vi "Color Threshold Handler.vi"(8 "error in (no error)":errorcluster, 11 "Range Updater Cntrl in":T1) -> (0 "error out":errorcluster, 3 "Range Updater Cntrl out":T1)   [LabVIEW 2018]
uses:
  Shared Controls/Range Updater.ctl
  Shared Controls/Threshold Updater.ctl
  Val Change Checker.vi
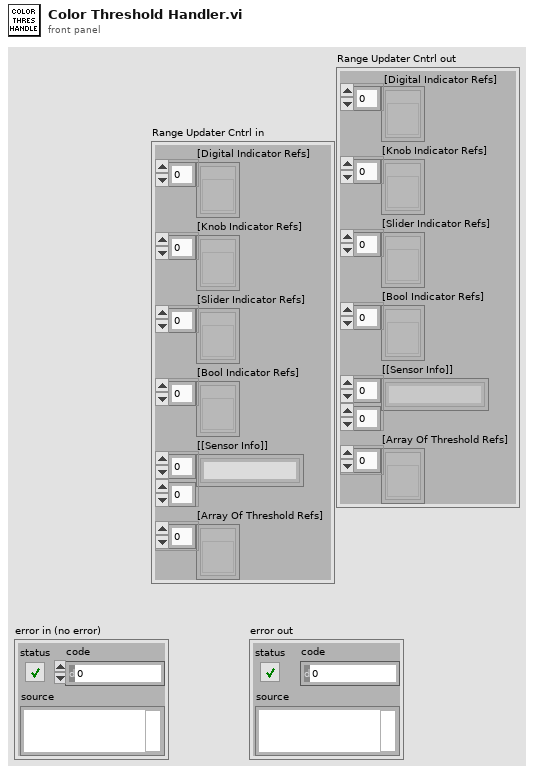
[diagram p1: front panel]
types:
  T1 = typedef "Range Updater.ctl" = cluster{"[Digital Indicator Refs]":refnum<vi>[], "[Knob Indicator Refs]":refnum<vi>[], "[Slider Indicator Refs]":refnum<vi>[], "[Bool Indicator Refs]":refnum<vi>[], "[[Sensor Info]]":string[][], "[Array Of Threshold Refs]":refnum<vi>[]}
  T2 = typedef "Threshold Updater.ctl" = cluster{"Red Min":dbl, "Yellow Min":dbl, "Yellow Max":dbl, "Red Max":dbl}
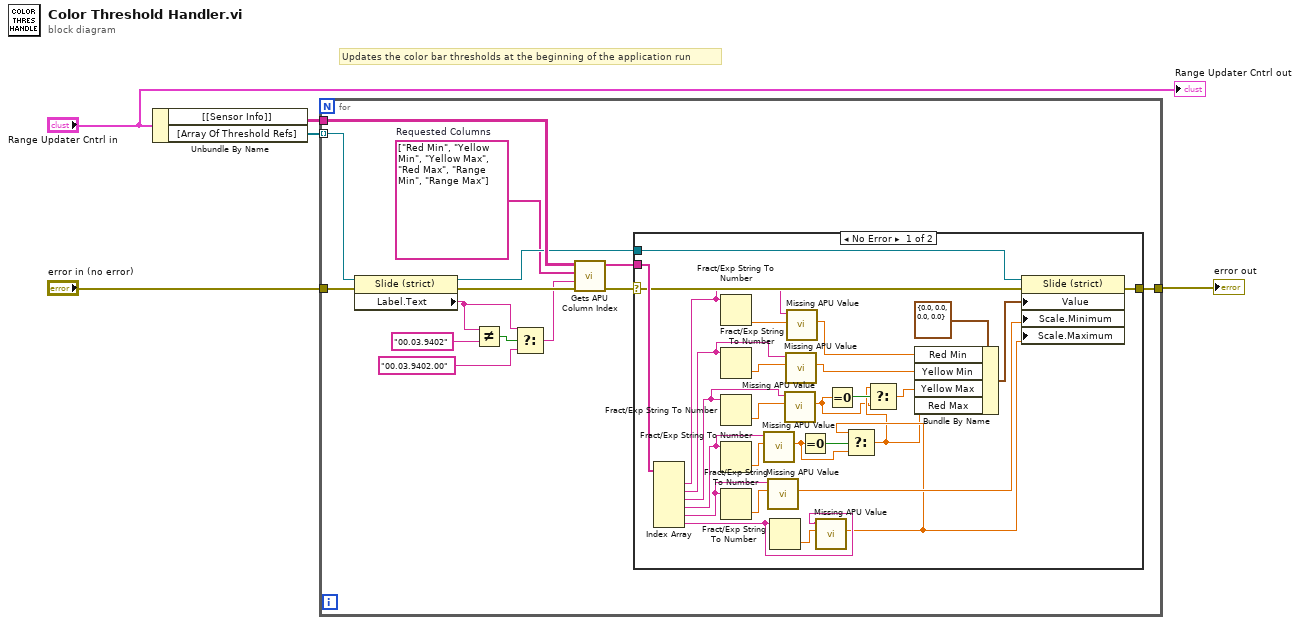
[diagram p0: block diagram]
diagram:
  # "Updates the color bar thresholds at the beginning of the application run"
  n1 = Unbundle By Name("Range Updater Cntrl in") -> ("[[Sensor Info]]"=w3:string[][], "[Array Of Threshold Refs]"=w2:refnum<vi>[])
  n2 = for {
    tunnel: w2 -> [w19] mode=indexing
    tunnel: "error in (no error)" -> [w18]
    tunnel: w3 -> [w15]
    tunnel: [w16] -> w4
    w13 = string[] ["Red Min", "Yellow Min", "Yellow Max", "Red Max", "Range Min", "Range Max"]  # Requested Columns
    n3 = property class="Slide (strict)"(reference=w19, error in=w18) -> (reference out=w14:refnum<vi>, error out=w17:errorcluster, "Label.Text"=w8:string)
    n4 = Not Equal?(x=w8, y="00.03.9402") -> (x != y?=w9:bool)
    n5 = Select(t=w8, s=w9, f="00.03.9402.00" ("y")) -> (s? t:f=w6:string)
    n6 = call "Gets APU Column Index.vi"("error in (no error)"=w17, "Tag"=w6, "[Column Names]"=w13, "[[Array of Info]]"=w15) -> ("error out"=w12:errorcluster, "[Values out]"=w11:string[])  [unwired: 3 in, 3 out]
    n7 = case shown="No Error" w12 {
      selector: w12 -> [w44 w48]
      tunnel: [w47 w48] -> w16
      tunnel: w14 -> [w46 _]
      tunnel: w11 -> [w45 _]
      frame No Error {
        n8 = Index Array(array=w45) -> (element #1=w40:string, element #2=w37:string, element #3=w34:string, element #4=w31:string, element #5=w28:string, element #6=w25:string)  [unwired: 6 in]
        n9 = Fract/Exp String To Number(string=w40) -> (number=w41:dbl)  [unwired: 3 in, 1 out]
        n10 = Fract/Exp String To Number(string=w37) -> (number=w38:dbl)  [unwired: 3 in, 1 out]
        n11 = Fract/Exp String To Number(string=w34) -> (number=w35:dbl)  [unwired: 3 in, 1 out]
        n12 = Fract/Exp String To Number(string=w31) -> (number=w32:dbl)  [unwired: 3 in, 1 out]
        n13 = Fract/Exp String To Number(string=w28) -> (number=w29:dbl)  [unwired: 3 in, 1 out]
        n14 = call "Missing APU Value.vi"("Num In"=w32, "String In"=w31) -> ("Num Out"=w30:dbl)  [unwired: 7 in, 2 out]
        n15 = call "Missing APU Value.vi"("Num In"=w29, "String In"=w28) -> ("Num Out"=w27:dbl)  [unwired: 7 in, 2 out]
        n16 = Fract/Exp String To Number(string=w25) -> (number=w26:dbl)  [unwired: 3 in, 1 out]
        n17 = call "Missing APU Value.vi"("Num In"=w35, "String In"=w34) -> ("Num Out"=w21:dbl)  [unwired: 7 in, 2 out]
        n18 = call "Missing APU Value.vi"("Num In"=w38, "String In"=w37) -> ("Num Out"=w36:dbl)  [unwired: 7 in, 2 out]
        n19 = call "Missing APU Value.vi"("Num In"=w41, "String In"=w40) -> ("Num Out"=w39:dbl)  [unwired: 7 in, 2 out]
        n20 = Equal To 0?(x=w30) -> (x = 0?=w33:bool)
        n21 = call "Missing APU Value.vi"("Num In"=w26, "String In"=w25) -> ("Num Out"=w24:dbl)  [unwired: 7 in, 2 out]
        n22 = Equal To 0?(x=w21) -> (x = 0?=w23:bool)
        n23 = Select(t=w24, s=w33, f=w30) -> (s? t:f=w22:dbl)
        n24 = Select(t=w22, s=w23, f=w21) -> (s? t:f=w20:dbl)
        n25 = Bundle By Name(cluster=T2 {"Red Min"=0.0, "Yellow Min"=0.0, "Yellow Max"=0.0, "Red Max"=0.0} ("Value"), "Red Min"=w39, "Yellow Min"=w36, "Yellow Max"=w20, "Red Max"=w22) -> (w42:T2)
        n26 = property class="Slide (strict)"(reference=w46, error in=w44, "Value"=w42, "Scale.Minimum"=w27, "Scale.Maximum"=w24) -> (error out=w47:errorcluster)  [unwired: 1 out]
      }
      frame Error {
        # "A Column Requested was not found!"
      }
    }
  }
  "error out" <- w4
  "Range Updater Cntrl out" <- "Range Updater Cntrl in"
